vi "S2C_Access_Update.vi"(7 "Condition":string, 8 "Error In":errorcluster, 9 "Data":variant, 10 "Columns":string[](array[string]), 11 "Table":string) -> (0 "Error Out":errorcluster)   [LabVIEW 2015]
uses:
  S2C_Access_Globals.vi
  <vilib>/addons/database/NI_Database_API.lvlib
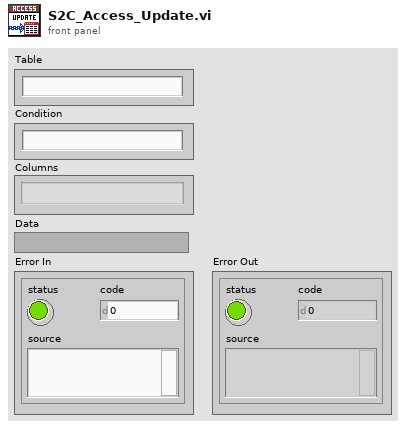
[diagram p1: front panel]
types:
  T1 = typedef "NI_Database_API.lvlib/Conn ObjectReference.ctl" = refnum<k1>
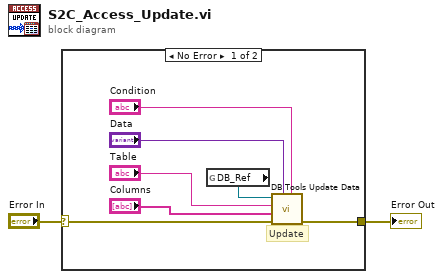
[diagram p0: block diagram]
diagram:
  n1 = case shown="No Error" "Error In" {
    selector: "Error In" -> [w9 w10]
    tunnel: [w8 w10] -> w1
    frame No Error {
      # "Update"
      n2 = global read "S2C_Access_Globals.vi" "DB_Ref"() -> (w7:T1)
      n3 = call <vilib>:"DB Tools Update Data.vi"("condition"="Condition", "data"="Data", "error in (no error)"=w9, "columns"="Columns", "table"="Table", "connection reference"=w7) -> ("error out"=w8:errorcluster)  [unwired: 4 in, 1 out]
    }
    frame Error {
    }
  }
  "Error Out" <- w1
